vi "V-Meter Measure.vi"(7 "Boolean":bool, 8 "error in (no error)":errorcluster, 11 "VISA resource name in":refnum<visa-resource-name>) -> (0 "error out":errorcluster, 2 "Measurement":dbl, 3 "VISA resource name out":refnum<visa-resource-name>)   [LabVIEW 2016, in "Hall Effect Library.lvlib"]
uses:
  Hall Effect Library.lvlib
  Global Variables/Instruments.vi
  V-Meter Measure (2000).vi
  V-Meter Measure (2182A).vi
  Global Variables/Test Settings.vi
  V-Meter Measure (3706).vi
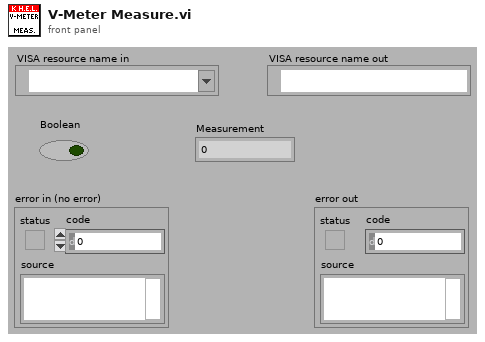
[diagram p1: front panel]
types:
  T1 = typedef "Hall Effect Library.lvlib/Voltmeters.ctl" = enum16{"2000", "2182A", "3706A"}
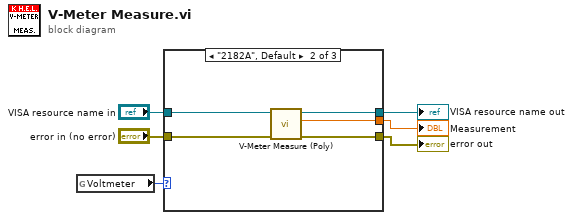
[diagram p0: block diagram]
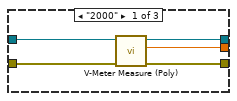
[diagram p2: hidden frame]
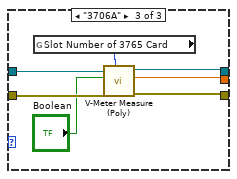
[diagram p3: hidden frame]
diagram:
  n1 = global read "Instruments.vi" "Voltmeter"() -> (w6:T1)
  n2 = case shown="\"2182A\", Default" w6 {
    tunnel: "error in (no error)" -> [w11 w16 w22]
    tunnel: "VISA resource name in" -> [w10 w15 w23]
    tunnel: [w9 w14 w21] -> w5
    tunnel: [w8 w13 w19] -> w3
    tunnel: [w7 w12 w20] -> w4
    frame "2000" {
      n3 = call-poly "V-Meter Measure (Poly).vi"("error in (no error)"=w11, "VISA resource name in"=w10) -> ("error out"=w8:errorcluster, "Measurement"=w7:dbl, "VISA resource name out"=w9:refnum<visa-resource-name>)  [unwired: 7 out]
    }
    frame "2182A", Default {
      n4 = call-poly "V-Meter Measure (Poly).vi"("error in (no error)"=w16, "VISA resource name in"=w15) -> ("error out"=w13:errorcluster, "Measurement"=w12:dbl, "VISA resource name out"=w14:refnum<visa-resource-name>)  [unwired: 7 out]
    }
    frame "3706A" {
      n5 = global read "Test Settings.vi" "Slot Number of 3765 Card"() -> (w18:u32)
      n6 = call-poly "V-Meter Measure (Poly).vi"("Slot Number"=w18, "error in (no error)"=w22, "Boolean"="Boolean", "VISA resource name in"=w23) -> ("error out"=w19:errorcluster, "Measurement"=w20:dbl, "VISA resource name out"=w21:refnum<visa-resource-name>)  [unwired: 5 in]
    }
  }
  "error out" <- w3
  "VISA resource name out" <- w5
  "Measurement" <- w4
